vi "Write Current Filter.vi"(8 "error in (no error)":errorcluster, 10 "Current Filter":u16(ring)=1 items=["Methane", "U", "B", "V", "R", "I", "Clear"], 11 "Roda_Filtros in":refnum<class "Roda_Filtros.lvclass">) -> (0 "error out":errorcluster, 3 "Roda_Filtros out":refnum<class "Roda_Filtros.lvclass">)   [LabVIEW 2018, in "Roda_Filtros.lvclass"]
uses:
  Roda_Filtros.lvclass
  Roda_Filtros.lvclass/Roda_Filtros.ctl
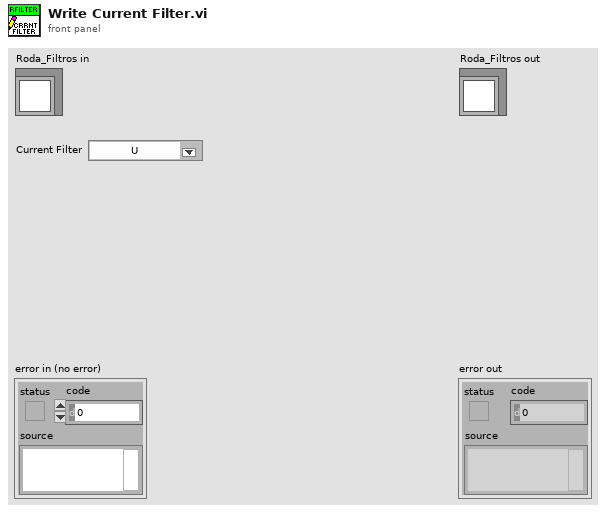
[diagram p1: front panel]
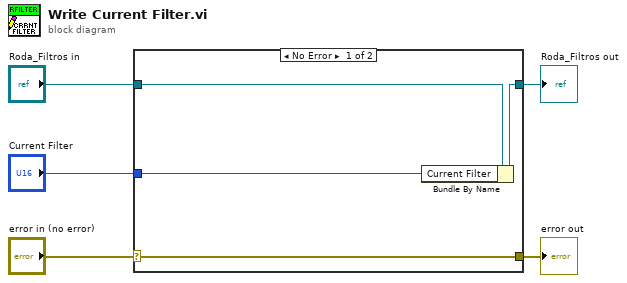
[diagram p0: block diagram]
diagram:
  n1 = case shown="No Error" "error in (no error)" {
    selector: "error in (no error)" -> [w9 w10]
    tunnel: [w9 w10] -> w4
    tunnel: [w7 w11] -> w2
    tunnel: "Roda_Filtros in" -> [w8 w11]
    tunnel: "Current Filter" -> [w6 _]
    frame No Error {
      n2 = Bundle By Name(cluster=w8, "Current Filter"=w6) -> (w7:refnum<class "Roda_Filtros.lvclass">)
    }
    frame Error {
    }
  }
  "error out" <- w4
  "Roda_Filtros out" <- w2
